vi "Weighted_Fast_Response_Stats.vi"(0 "U":dbl[](array[numeric]) format="%.2f", 1 "Index":i32, 5 "Weighting":dbl[](array[numeric]) format="%.2f", 11 "Shift in":dbl[](array[numeric]) format="%.2f", 12 "Block No":i32=1) -> (4 "Results file string array":string[](array[string]), 15 "Shift out":dbl[](array[numeric]) format="%.2f")   [LabVIEW 2010]
uses:
  Globals/Meas_global.vi
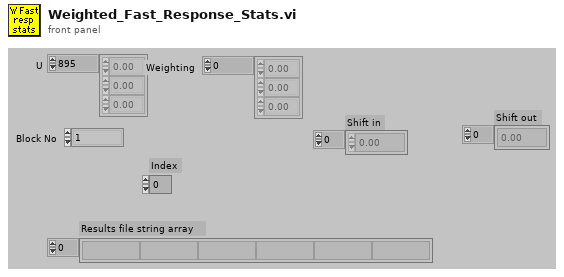
[diagram p1: front panel]
types:
  T1 = typedef "Velocity_cluster.ctl" = cluster{"Name":string, "U":dbl, "u^2":dbl, "u^3/(u^2)^(1.5)":dbl, "u^4/(u^2)^2 -3":dbl, "% u'/U":dbl, "Mean % Err":dbl, "u^4":dbl}
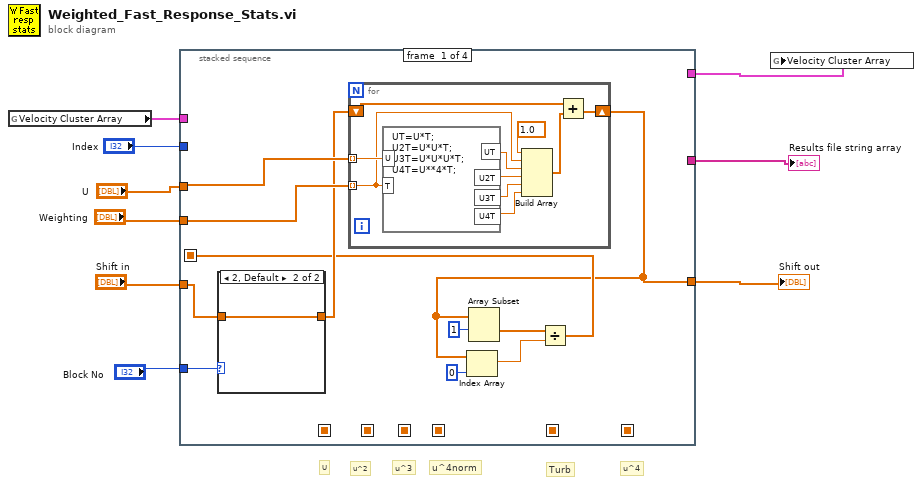
[diagram p0: block diagram]
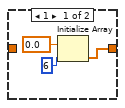
[diagram p2: hidden frame]
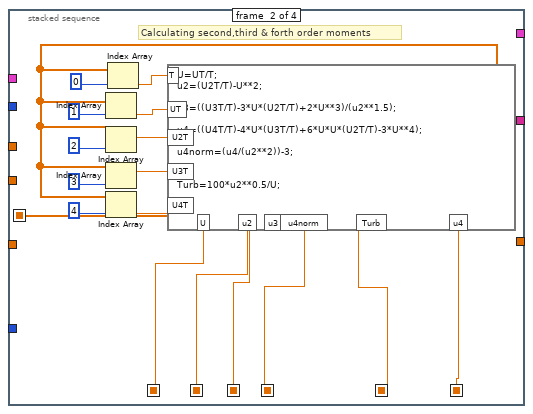
[diagram p3: hidden frame]
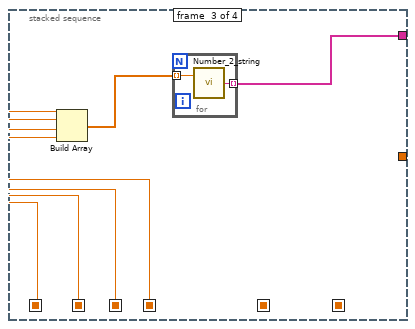
[diagram p4: hidden frame]
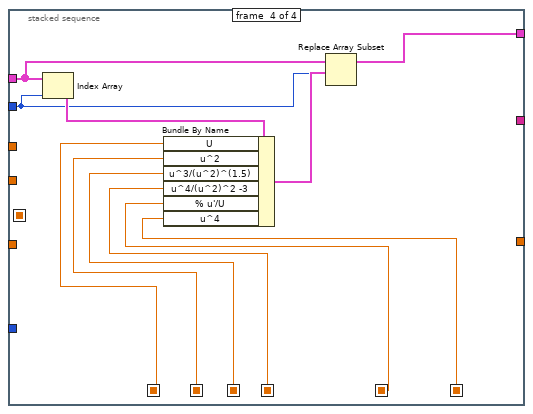
[diagram p5: hidden frame]
diagram:
  # "u^4"
  # "u^4norm"
  # "u^3"
  # "Turb"
  # "U"
  # "u^2"
  n1 = global read "Meas_global.vi" "Velocity Cluster Array"() -> (w6:T1[])
  n2 = stacked-sequence {
    seq-local: [_ w48 _ _] -> [_ _ w56 w64]
    seq-local: [w11 _ _ _] -> [_ w45 _ _]
    seq-local: [_ w46 _ _] -> [_ _ w57 w65]
    seq-local: [_ w49 _ _] -> [_ _ _ w63]
    seq-local: [_ w37 _ _] -> [_ _ w55 w62]
    seq-local: [_ w36 _ _] -> [_ _ w54 w61]
    seq-local: [_ w35 _ _] -> [_ _ _ w60]
    tunnel: "U" -> [w20 _ _ _]
    tunnel: [w10 _ _ _] -> w8
    tunnel: "Shift in" -> [w13 _ _ _]
    tunnel: [_ _ w52 _] -> w7
    tunnel: w6 -> [_ _ _ w68]
    tunnel: "Index" -> [_ _ _ w67]
    tunnel: [_ _ _ w66] -> w4
    tunnel: "Weighting" -> [w19 _ _ _]
    tunnel: "Block No" -> [w14 _ _ _]
    frame #0 {
      n3 = case shown="2, Default" w14 {
        tunnel: [w21 w24] -> w12
        tunnel: w13 -> [_ w24]
        frame 1 {
          n4 = Initialize Array(0.0 ("Element Data"), 6 ("Dimension Size")) -> (w21:dbl[])
        }
        frame 2, Default {
        }
      }
      n5 = for {
        shift-right: [w33] -> w10
        shift-left: w12 -> [w34]
        tunnel: w20 -> [w31] mode=indexing
        tunnel: w19 -> [w30] mode=indexing
        n6 = formula code="UT=U*T;\nU2T=U*U*T;\nU3T=U*U*U*T;\nU4T=U**4*T;"("U"=w31, "T"=w30) -> ("U2T"=w28:dbl, "UT"=w29:dbl, "U3T"=w27:dbl, "U4T"=w26:dbl)
        n7 = Build Array(1.0 ("Input Element"), w30, w29, w28, w27, w26) -> (w32:dbl[])
        n8 = Add(x=w34, y=w32) -> (x+y=w33:dbl[])
      }
      n9 = Index Array(array=w10, index=0 ("Index")) -> (element=w15:dbl)
      n10 = Array Subset(array=w10, index=1 ("Array Index")) -> (w16:dbl[])  [unwired: 1 in]
      n11 = Divide(x=w16, y=w15) -> (x/y=w11:dbl[])
    }
    frame #1 {
      # "Calculating second,third & forth order moments"
      n12 = Index Array(array=w45, index=1) -> (element=w41:dbl)
      n13 = Index Array(array=w45, index=2) -> (element=w40:dbl)
      n14 = Index Array(array=w45, index=3) -> (element=w39:dbl)
      n15 = Index Array(array=w45, index=4) -> (element=w38:dbl)
      n16 = Index Array(array=w45, index=0) -> (element=w42:dbl)
      n17 = formula code="U=UT/T;\nu2=(U2T/T)-U**2;\n\nu3=((U3T/T)-3*U*(U2T/T)+2*U**3)/(u2**1.5);\n\nu4=((U4T/T)-4*U*(U3T/T)+6*U*U*(U2T/T)-3*U**4);\n\nu4norm=(u4/(u2**2))-3;\n\n\nTurb=100*u2**0.5/U;"("T"=w42, "UT"=w41, "U2T"=w40, "U3T"=w39, "U4T"=w38) -> ("u2"=w48:dbl, "Turb"=w49:dbl, "U"=w46:dbl, "u3"=w37:dbl, "u4"=w35:dbl, "u4norm"=w36:dbl)
    }
    frame #2 {
      n18 = Build Array(w57, w56, w55, w54) -> (w53:dbl[])
      n19 = for {
        tunnel: w53 -> [w59] mode=indexing
        tunnel: [w58] -> w52 mode=indexing
        n20 = call "Number_2_string.vi"("number"=w59) -> ("String"=w58:string)  [unwired: 1 in]
      }
    }
    frame #3 {
      n21 = Index Array(array=w68, index=w67) -> (element=w70:T1)
      n22 = Bundle By Name(cluster=w70, "U"=w65, "u^2"=w64, "u^3/(u^2)^(1.5)"=w62, "u^4/(u^2)^2 -3"=w61, "% u'/U"=w63, "u^4"=w60) -> (w69:T1)
      n23 = Replace Array Subset(array=w68, new element=w69, index=w67) -> (w66:T1[])
    }
  }
  "Shift out" <- w8
  "Results file string array" <- w7
  n24 = global write "Meas_global.vi" "Velocity Cluster Array"(w4) -> ()
